vi "Write acquisition configuration.vi"(8 "error in (no error)":errorcluster, 11 "Channel in":refnum<class "Channel.lvclass">) -> (0 "error out":errorcluster, 3 "Channel out":refnum<class "Channel.lvclass">)   [LabVIEW 2018, in "Channel.lvclass"]
uses:
  Channel.lvclass
  Channel.lvclass/Channel.ctl
  Simulated_CCD_Camera/Simulated_CCD_Camera.lvclass/Simulated_CCD_Camera.ctl
  Simulated_CCD_Camera/Simulated_CCD_Camera.lvclass
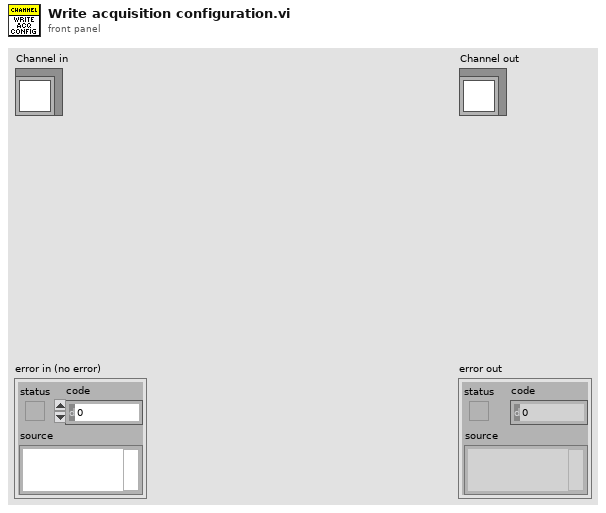
[diagram p1: front panel]
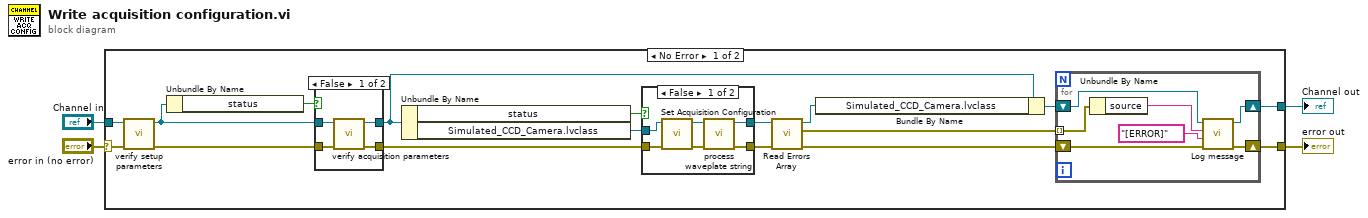
[diagram p0: block diagram]
diagram:
  n1 = case shown="No Error" "error in (no error)" {
    selector: "error in (no error)" -> [w8 w44]
    tunnel: [w10 w44] -> w3
    tunnel: [w11 w43] -> w1
    tunnel: "Channel in" -> [w9 w43]
    frame No Error {
      n2 = call "verify setup parameters.vi"("error in (no error)"=w8, "Channel in"=w9) -> ("error out"=w7:errorcluster, "Channel out"=w6:refnum<class "Channel.lvclass">)  [unwired: 8 in]
      n3 = Unbundle By Name(w6) -> ("status"=w5:bool)
      n4 = case shown="False" w5 {
        tunnel: [w25 w27] -> w13
        tunnel: [w24 w26] -> w12
        tunnel: w7 -> [w23 w26]
        tunnel: w6 -> [w22 w27]
        frame False {
          n5 = call "verify acquisition parameters.vi"("error in (no error)"=w23, "Channel in"=w22) -> ("error out"=w24:errorcluster, "Channel out"=w25:refnum<class "Channel.lvclass">)  [unwired: 8 in]
        }
        frame True {
        }
      }
      n6 = Unbundle By Name(w13) -> ("status"=w21:bool, "Simulated_CCD_Camera.lvclass"=w20:refnum<class "Simulated_CCD_Camera.lvclass">)
      n7 = case shown="False" w21 {
        tunnel: w20 -> [w39 w42]
        tunnel: w12 -> [w40 w41]
        tunnel: [w38 w41] -> w19
        tunnel: [w37 w42] -> w14
        frame False {
          n8 = call-dynamic "Set Acquisition Configuration.vi"("error in (no error)"=w40, "CCDCamera in"=w39) -> ("error out"=w35:errorcluster, "CCDCamera out"=w36:refnum<class "Simulated_CCD_Camera.lvclass">)  [unwired: 8 in]
          n9 = call "process waveplate string.vi"("error in (no error)"=w35, "Simulated_CCD_Camera in"=w36) -> ("error out"=w38:errorcluster, "Simulated_CCD_Camera out"=w37:refnum<class "Simulated_CCD_Camera.lvclass">)  [unwired: 8 in]
        }
        frame True {
        }
      }
      n10 = call "Read Errors Array.vi"("error in (no error)"=w19, "Simulated_CCD_Camera in"=w14) -> ("error out"=w15:errorcluster, "Errors array"=w16:errorcluster[], "Simulated_CCD_Camera out"=w18:refnum<class "Simulated_CCD_Camera.lvclass">)  [unwired: 7 in]
      n11 = Bundle By Name(cluster=w13, "Simulated_CCD_Camera.lvclass"=w18) -> (w17:refnum<class "Channel.lvclass">)
      n12 = for {
        shift-right: [w33] -> w11
        shift-left: w17 -> [w34]
        shift-right: [w32] -> w10
        shift-left: w15 -> [w30]
        tunnel: w16 -> [w29] mode=indexing
        n13 = Unbundle By Name(w29) -> ("source"=w28:string)
        n14 = call "Log message.vi"("error in (no error)"=w30, "message type"="[ERROR]", "String"=w28, "Channel in"=w34) -> ("error out"=w32:errorcluster, "Channel out"=w33:refnum<class "Channel.lvclass">)  [unwired: 6 in]
      }
    }
    frame Error {
    }
  }
  "error out" <- w3
  "Channel out" <- w1
